vi "Sensor - Fire Deposit.vi"(8 "error in (no error)":errorcluster, 10 "Deposit Received":bool, 11 "View Model":T1) -> (0 "error out":errorcluster, 3 "View Model":T1)   [LabVIEW 2017]
doc: "Generate user Event for Received Deposit."
uses:
  View Model/Controls/View Model.ctl
  View Model/Controls/Shared Model.ctl
  Error Handler/Controls/Error Model.ctl
  Error Handler/Controls/Error Data.ctl
  Error Handler/Controls/Error Type.ctl
  Error Handler/Controls/Error Source.ctl
  Configuration/Controls/Config Model.ctl
  Configuration/Controls/Config CMD.ctl
  Configuration/Controls/Config Command.ctl
  Controller/Controls/Controller Model.ctl
  Controller/Controls/Controller Overhead.ctl
  Controller/Controls/Controller Transaction.ctl
  Controller/Controls/Controller State.ctl
  Configuration/Controls/Config Data Record.ctl
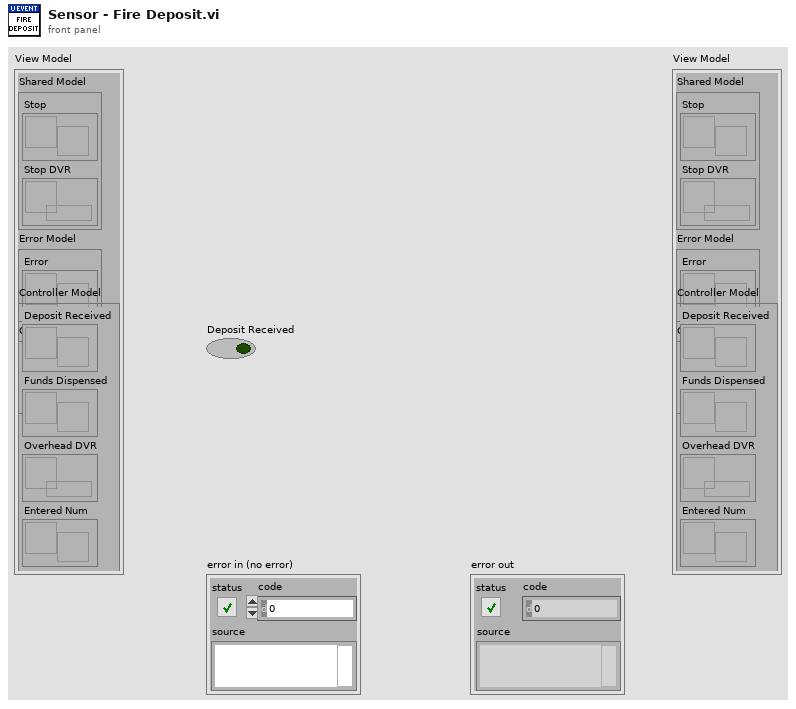
[diagram p1: front panel]
types:
  T1 = typedef "View Model.ctl" = cluster{"Shared Model":T2, "Error Model":T3, "Config Model":T4, "Controller Model":T5}
  T2 = typedef "Shared Model.ctl" = cluster{"Stop":refnum<user-event>, "Stop DVR":refnum<data-value>}
  T3 = typedef "Error Model.ctl" = cluster{"Error":refnum<user-event>}
  T4 = typedef "Config Model.ctl" = cluster{"Config CMD":refnum<user-event>}
  T5 = typedef "Controller Model.ctl" = cluster{"Deposit Received":refnum<user-event>, "Funds Dispensed":refnum<user-event>, "Overhead DVR":refnum<data-value>, "Entered Num":refnum<user-event>, "Card Read":refnum<user-event>, "Transaction":refnum<user-event>}
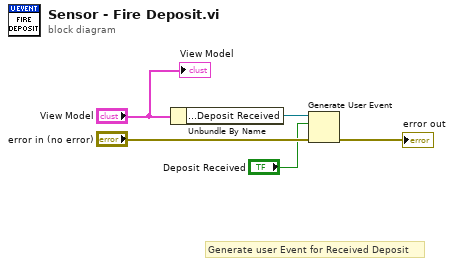
[diagram p0: block diagram]
diagram:
  # "Generate user Event for Received Deposit"
  n1 = Unbundle By Name("View Model") -> ("Controller Model.Deposit Received"=w5:refnum<user-event>)
  n2 = Generate User Event(user event=w5, event data cluster="Deposit Received", error in="error in (no error)") -> (error out=→"error out":errorcluster)  [unwired: 1 in, 1 out]
  "View Model" <- "View Model"
